vi "AMX-CCD3 自动处理图像 - 副本 - 副本.vi"(0 "Image IN":T1(plugin-control), 9 "A/B段位置切换":bool, 11 "error in (no error)":errorcluster caption="错误输入（无错误）") -> (4 "Image Out":T1(plugin-control), 6 "结果":bool, 10 "颗粒物有无判断":bool, 14 "结果数组":bool[](array[boolean]), 15 "error out":errorcluster caption="错误输出")   [LabVIEW 2017]
uses:
  Global System.vi
panel:
  out "Number of Features Found":i32
  in  "颗粒物个数阈值":i32
  out "颗粒物大小显示":dbl[](array[numeric])
  out "颗粒物位置坐标":cluster{"X":dbl, "Y":dbl}[](array[cluster]) {"Y" format="%.2f"; "X" format="%.2f"}
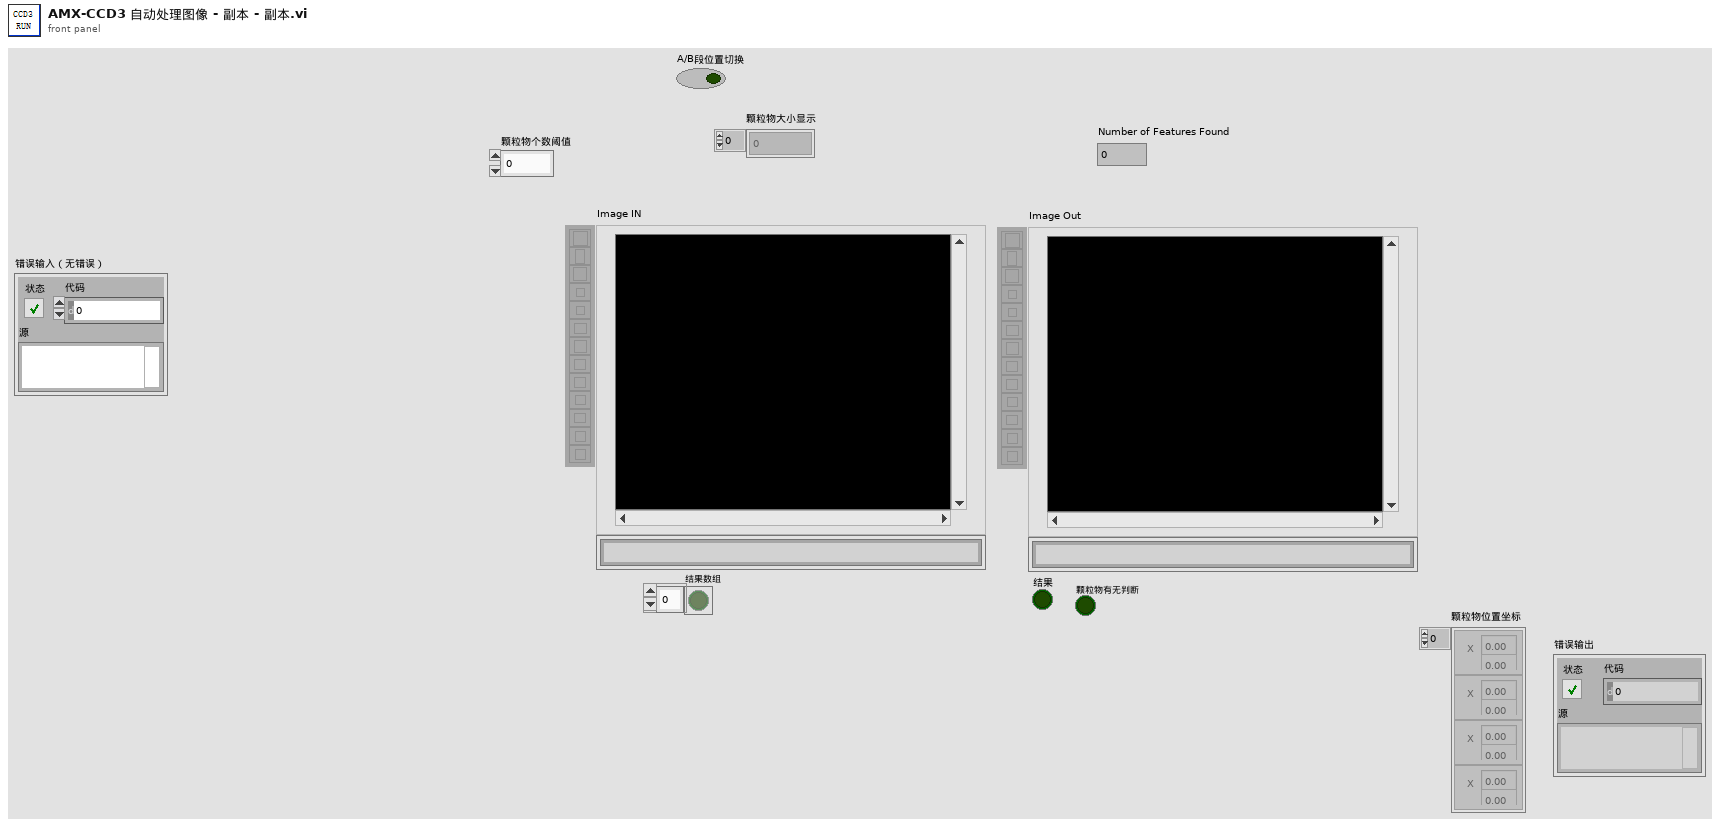
[diagram p1: front panel]
types:
  T1 = typedef "IMAQ Image.ctl" = refnum<image>
  T2 = typedef "Image Type" = u32
  T3 = typedef "IMAQ Rectangle" = cluster{"Left":i32, "Top":i32, "Right":i32, "Bottom":i32, "Rotation":dbl}
  T4 = cluster{"Rectangle":T3, "Threshold Limits (Threshold 1)":cluster{"Lower value":sgl, "Upper value":sgl}, "Keep/Remove Particles ":bool, "Connectivity 4/8 (8) ":bool, "Selection Values (Particle Filter 1)":cluster{"Measurement Parameter":i32, "Range Lower Value":dbl, "Range Upper Value":dbl, "Range":bool, "Measurement Type":bool}[], "Corner Options (Feature Detection 1)":cluster{"Detector type":enum32{"Harris Corner", "Shi-Tomasi Corner"}, "Kernel size":i32, "Min Corner Point Strength":dbl}, "Pyramid level (Feature Detection 1)":u32, "Method ":i32, "Look For":u32, "Method 2":i32, "ROI Descriptor (Clamp (Rake) 1)":cluster{"Global Rectangle":i32[], "Contours":cluster{"ID":enum32{"External", "Internal"}, "Type":u32, "Coordinates":i32[]}[]}}
  T5 = typedef "IMAQ Curve Parameters.ctl" = cluster{"Extraction Mode":u32, "Edge Threshold":i32, "Edge Filter Size":u32, "Min Length":i32, "Row Search Step Size":i32, "Col Search Step Size":i32, "Max Endpoint Gap":i32, "Closed":bool, "Subpixel":bool}
  T6 = cluster{"Max Number":sgl, "Curve Extraction Settings ":T5, "Color Mode (Histogram 1)":u16, "Range (Threshold 1)":cluster{"Lower value":sgl, "Upper value":sgl}, "Clamp Settings (Max Clamp 1)":cluster{"Angle Range (+/-)":dbl, "Edge Polarity":cluster{"Start":u32, "End":u32}}, "Settings (Clamp (Rake) 1)":cluster{"Contrast":i32, "Filter width":i32, "Steepness":i32, "Subsampling Ratio":u32, "Show Search Area":bool, "Show Search Lines":bool, "Show Edges Found":bool, "Show Result":bool}}
  T7 = typedef "IMAQdx.ctl" = refnum<k21>
  T8 = cluster{"IsNorImage":bool, "Exposure Values":u32, "ImagePath":path, "相机选择":T7}
  T9 = cluster{"Desired Font (Application)":enum16{"User-specified Font", "Application Font", "System Font", "Dialog Font"}, "[User-specified Font]":cluster{"Font Name":string, "Size":i16, "Strikeout?":bool, "Italic?":bool, "Underline?":bool, "Outline?":bool, "Shadow?":bool, "Bold?":bool, "Rotation Angle":dbl}, "Horizontal Alignment":i16, "Vertical Alignment":i16}
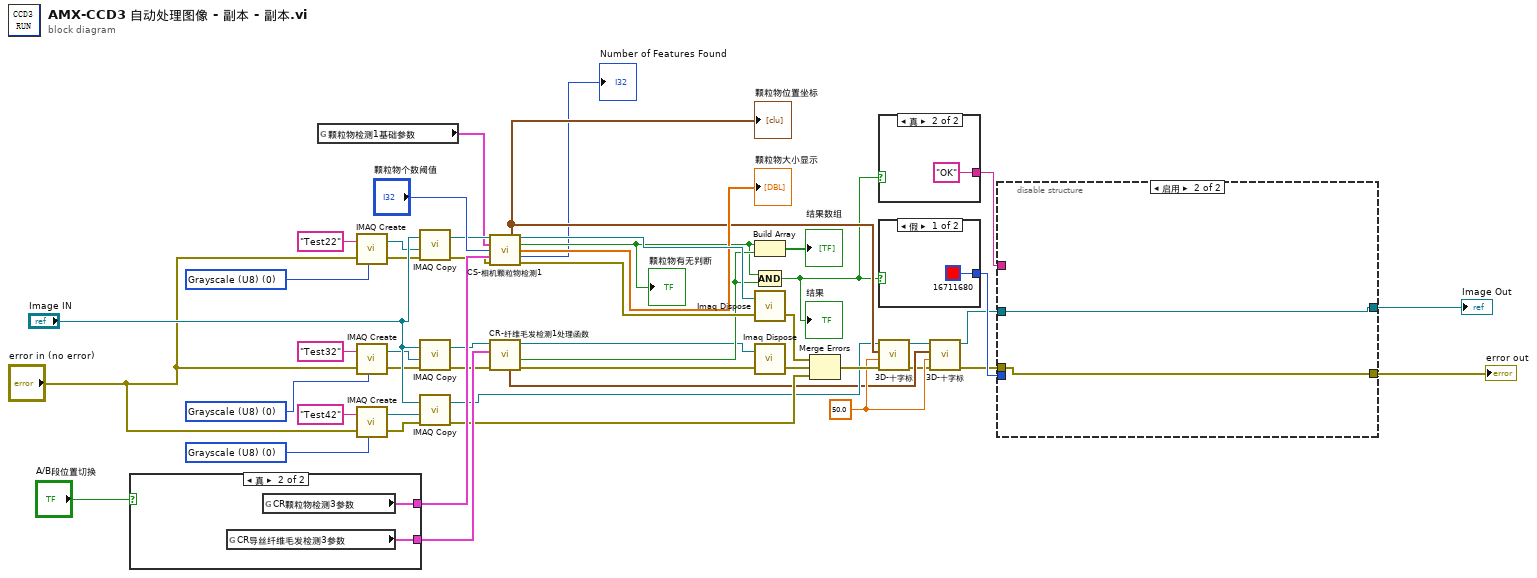
[diagram p0: block diagram]
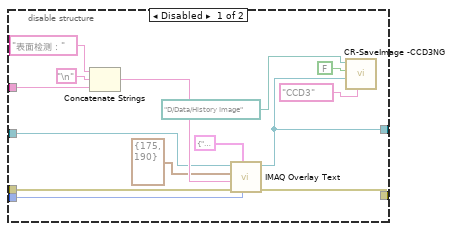
[diagram p2: hidden frame]
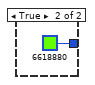
[diagram p3: hidden frame]
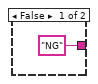
[diagram p4: hidden frame]
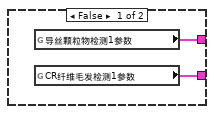
[diagram p5: hidden frame]
diagram:
  w18 = 50.0 ("radius")
  w32 = T2 0 items=["Grayscale (U8)", "Grayscale (I16)", "Grayscale (SGL)", "Complex (CSG)", "RGB (U32)", "HSL (U32)", "RGB (U64)", "Grayscale (U16)"] ("Image Type")
  w34 = T2 0 items=["Grayscale (U8)", "Grayscale (I16)", "Grayscale (SGL)", "Complex (CSG)", "RGB (U32)", "HSL (U32)", "RGB (U64)", "Grayscale (U16)"] ("Image Type")
  w39 = T2 0 items=["Grayscale (U8)", "Grayscale (I16)", "Grayscale (SGL)", "Complex (CSG)", "RGB (U32)", "HSL (U32)", "RGB (U64)", "Grayscale (U16)"] ("Image Type")
  n1 = case shown="真" "A/B段位置切换" {
    tunnel: [w51 w53] -> w44
    tunnel: [w50 w52] -> w43
    frame False {
      n2 = global read "Global System.vi" "导丝颗粒物检测1参数"() -> (w51:T4)
      n3 = global read "Global System.vi" "CR纤维毛发检测1参数"() -> (w50:T6)
    }
    frame True {
      n4 = global read "Global System.vi" "CR导丝纤维毛发检测3参数"() -> (w52:T6)
      n5 = global read "Global System.vi" "CR颗粒物检测3参数"() -> (w53:T4)
    }
  }
  n6 = global read "Global System.vi" "颗粒物检测1基础参数"() -> (w15:T8)
  n7 = call "IMAQ Create"("Image Name"="Test22", "Image Type"=w39, "error in (no error)"="error in (no error)") -> ("New Image"=w29:T1, "error out"=w27:errorcluster)  [unwired: 2 in]
  n8 = call "IMAQ Create"("Image Name"="Test32", "Image Type"=w32, "error in (no error)"="error in (no error)") -> ("New Image"=w1:T1, "error out"=w4:errorcluster)  [unwired: 2 in]
  n9 = call "IMAQ Create"("Image Name"="Test42", "Image Type"=w34, "error in (no error)"="error in (no error)") -> ("New Image"=w25:T1, "error out"=w23:errorcluster)  [unwired: 2 in]
  n10 = call "IMAQ Copy"("error in (no error)"=w27, "Image Dst"=w29, "Image Src"="Image IN") -> ("error out"=w26:errorcluster, "Image Dst Out"=w28:T1)  [unwired: 3 in]
  n11 = call "IMAQ Copy"("error in (no error)"=w4, "Image Dst"=w1, "Image Src"="Image IN") -> ("error out"=w3:errorcluster, "Image Dst Out"=w2:T1)  [unwired: 3 in]
  n12 = call "IMAQ Copy"("error in (no error)"=w23, "Image Dst"=w25, "Image Src"="Image IN") -> ("error out"=w24:errorcluster, "Image Dst Out"=w20:T1)  [unwired: 3 in]
  n13 = call "CS-相机颗粒物检测1.vi"("Image in"=w28, "相机颗粒物检测1基础参数"=w15, "颗粒物个数阈值"="颗粒物个数阈值", "导丝颗粒物检测1参数"=w44, "error in (no error)"=w26) -> ("颗粒物位置坐标"=w21:cluster{"X":dbl, "Y":dbl}[], "Image out"=w38:T1, "颗粒物有无显示"=w19:bool, "颗粒物大小显示"=→"颗粒物大小显示":dbl[], "Number of Features Found"=→"Number of Features Found":i32, "error out"=w37:errorcluster)  [unwired: 4 in, 1 out]
  "颗粒物有无判断" <- w19
  "颗粒物位置坐标" <- w21
  n14 = call "CR-纤维毛发检测1处理函数.vi"("error in (no error)"=w3, "UI电源线正面漏线参数"=w43, "Image in"=w2) -> ("error out"=w6:errorcluster, "纤维毛发"=w30:bool, "Image out"=w7:T1, "Edge Coordinates (calibrated) (Clamp (Rake) 1)"=w17:cluster{"X":sgl, "Y":sgl}[])  [unwired: 4 in, 1 out]
  n15 = Build Array(w19, w30) -> (→"结果数组":bool[])
  n16 = call "Imaq Dispose"("Image"=w38, "error in (no error)"=w37) -> ("error out"=w40:errorcluster)  [unwired: 4 in]
  n17 = call "Imaq Dispose"("Image"=w7, "error in (no error)"=w6) -> ("error out"=w41:errorcluster)  [unwired: 4 in]
  n18 = Compound Arithmetic op=AND ("复合运算")(w19, w30) -> (w16:bool)
  "结果" <- w16
  n19 = Merge Errors(w40, w41, w24) -> (w22:errorcluster)
  n20 = case shown="真" w16 {
    tunnel: ["NG" "OK"] -> w10
    frame False {
    }
    frame True {
    }
  }
  n21 = case shown="假" w16 {
    tunnel: [u32 16711680 ("Text Color (black)") u32 6618880 ("Text Color (black)")] -> w11
    frame False {
    }
    frame True {
    }
  }
  n22 = call "3D-十字标.vi"("error in (no error)"=w22, "radius"=w18, "颗粒物位置坐标"=w21, "输入图片"=w20) -> ("error out"=w12:errorcluster, "输出图片"=w13:T1)  [unwired: 6 in]
  n23 = call "3D-十字标.vi"("error in (no error)"=w12, "radius"=w18, "颗粒物位置坐标"=w17, "输入图片"=w13) -> ("error out"=w8:errorcluster, "输出图片"=w9:T1)  [unwired: 6 in]
  n24 = disable-structure shown="启用" {
    disable-tunnel: [w71 w72] -> w47
    disable-tunnel: [w70 w73] -> w46
    disable-tunnel: w11 -> [w64 _]
    disable-tunnel: w10 -> [w61 _]
    disable-tunnel: w9 -> [w59 w73]
    disable-tunnel: w8 -> [w58 w72]
    frame Disabled {
      n25 = Concatenate Strings("表面检测：" ("字符串"), "\n", w61) -> (w66:string)
      n26 = call "IMAQ Overlay Text"("Text Color (black)"=w64, "Font, Size & Style"=T9 {"Desired Font (Application)"=enum."User-specified Font", "[User-specified Font]"={"Font Name"="", "Size"=100, "Strikeout?"=FALSE, "Italic?"=FALSE, "Underline?"=FALSE, "Outline?"=FALSE, "Shadow?"=FALSE, "Bold?"=FALSE, "Rotation Angle"=0.0}, "Horizontal Alignment"=0, "Vertical Alignment"=0}, "error in (no error)"=w58, "String"=w66, "Origin"=cluster{"X":i32, "Y":i32} {"X"=175, "Y"=190}, "Image"=w59) -> ("error out"=w71:errorcluster, "Image Out"=w70:T1)  [unwired: 4 in]
      n27 = call "CR-SaveImage -CCD3NG.vi"("CCD Name"="CCD3", "Image in"=w70, "布尔"=FALSE, "基路径"=path "D:/Data/History Image") -> ()  [unwired: 7 in, 1 out]
    }
    frame Enabled {
    }
  }
  "error out" <- w47
  "Image Out" <- w46
